vi "arduino write.vi"() -> ()   [LabVIEW 2014]
uses:
  <vilib>/Instr/_visa.llb/VISA Configure Serial Port (Instr).vi
panel:
  in  "stop":bool
  out "read buffer":string
  out "Waveform Chart":dbl(graph)
  in  "VISA resource name":refnum<visa-resource-name>
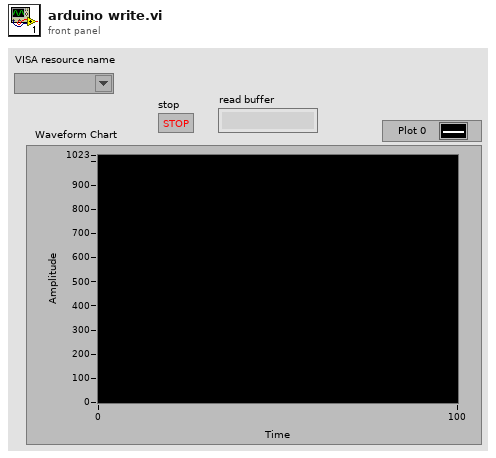
[diagram p1: front panel]
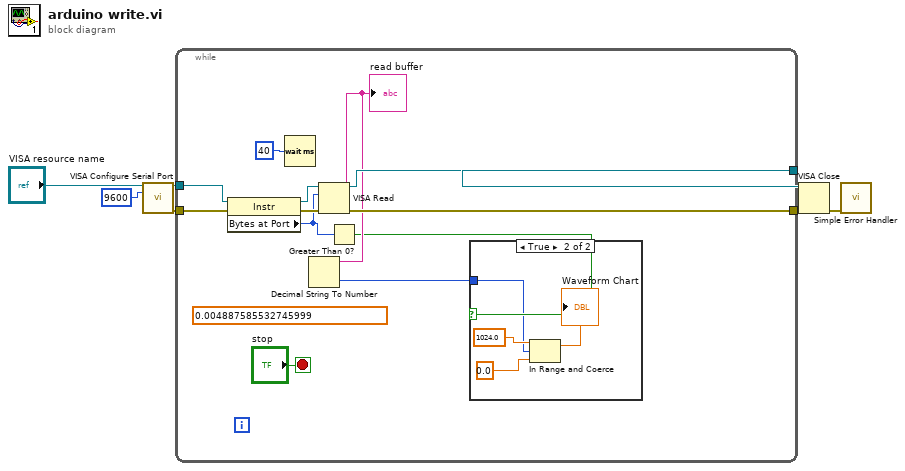
[diagram p0: block diagram]
diagram:
  n1 = call-poly "VISA Configure Serial Port"("VISA resource name"="VISA resource name", "baud rate (9600)"=u32 9600) -> ("VISA resource name out"=w5:refnum<visa-resource-name>, "error out"=w4:errorcluster)  [unwired: 12 in]
  n2 = while {
    tunnel: w5 -> [w19]
    tunnel: w4 -> [w18]
    tunnel: [w14] -> w3
    tunnel: [w15] -> w2
    stop <- "stop" stop-if-true
    (unwired) 0.004887585532745999
    n3 = property class="Instr"(reference=w19, error in=w18) -> (reference out=w13:refnum<visa-resource-name>, error out=w16:errorcluster, "Bytes at Port"=w10:u32)
    n4 = Wait (ms)(milliseconds to wait=u32 40) -> ()  [unwired: 1 out]
    n5 = VISA Read(VISA resource name=w13, byte count=w10, error in (no error)=w16) -> (VISA resource name out=w14:refnum<visa-resource-name>, read buffer=w12:string, error out=w15:errorcluster)  [unwired: 1 out]
    "read buffer" <- w12
    n6 = Decimal String To Number(string=w12) -> (number=w8:i32)  [unwired: 2 in, 1 out]
    n7 = Greater Than 0?(x=w10) -> (x > 0?=w9:bool)
    n8 = case shown="True" w9 {
      tunnel: w8 -> [_ w21]
      frame False {
      }
      frame True {
        n9 = In Range and Coerce(upper limit=1024.0, x=w21, lower limit=0.0) -> (coerced(x)=→"Waveform Chart":dbl)  [unwired: 1 out]
      }
    }
  }
  n10 = VISA Close(VISA resource name=w3, error in (no error)=w2) -> (error out=w1:errorcluster)
  n11 = call <vilib>:"Simple Error Handler.vi"("error in (no error)"=w1) -> ()  [unwired: 4 in, 5 out]
